vi "Teleop.vi"(10 "Match Info":T1={"Autonomous Elapsed Seconds"=0.0, "TeleOp Elapsed Seconds"=0.0, "Disabled Elapsed Seconds"=0.0, "Visited Autonomous"=FALSE, "Visited TeleOp"=FALSE, "Visited Disabled"=FALSE, "Autonomous Settings"={"Autonomous Style"=enum."Independent", "VI Refnum"=refnum}}, 11 "Call Context":T2) -> ()   [LabVIEW 2013]
doc: "This VI is called for each TeleOp packet received from the DS where the robot is not disabled. It is often used to read from the joysticks and update I/O or to update setpoints for timed control loops. It should complete and return within 20 milliseconds or it may miss DS packets."
uses:
  <vilib>/Rock Robotics/WPI/DriverStation/WPI_DriverStationDerivedRobotMode.ctl
  <vilib>/Rock Robotics/WPI/DriverStation/WPI_DriverStationMatch Info.ctl
  Robot Global Data.vi
  <vilib>/Rock Robotics/WPI/Joystick/WPI_JoystickGetSetRefNum.vi
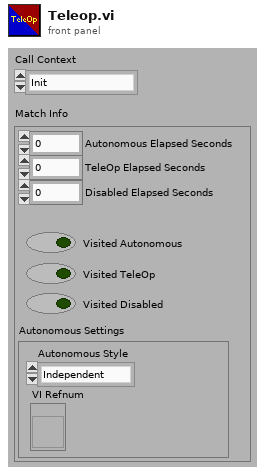
[diagram p1: front panel]
types:
  T1 = typedef "WPI_DriverStationMatch Info.ctl" = cluster{"Autonomous Elapsed Seconds":dbl, "TeleOp Elapsed Seconds":dbl, "Disabled Elapsed Seconds":dbl, "Visited Autonomous":bool, "Visited TeleOp":bool, "Visited Disabled":bool, "Autonomous Settings":cluster{"Autonomous Style":enum16{"Iterative", "Independent"}, "VI Refnum":refnum<vi>}}
  T2 = typedef "WPI_DriverStationDerivedRobotMode.ctl" = enum16{"Init", "Execute", "Stop"}
  T3 = typedef "WPI_JoystickDevRef.ctl" = cluster{"Device":T4}
  T4 = typedef "WPI_JoystickDeviceEnum.ctl" = enum16{"USB 1", "USB 2", "USB 3", "USB 4", "Kinect 1", "Kinect 2"}
  T5 = typedef "WPI_JoystickButtonState.ctl" = cluster{"Button 1":bool, "Button 2":bool, "Button 3":bool, "Button 4":bool, "Button 5":bool, "Button 6":bool, "Button 7":bool, "Button 8":bool, "Button 9":bool, "Button 10":bool, "Button 11":bool, "Button 12":bool}
  T6 = cluster{"axis 1 (x)":dbl, "axis 2 (y)":dbl, "axis 3 (throttle)":dbl, "axis 4":dbl, "axis 5":dbl, "axis 6":dbl}
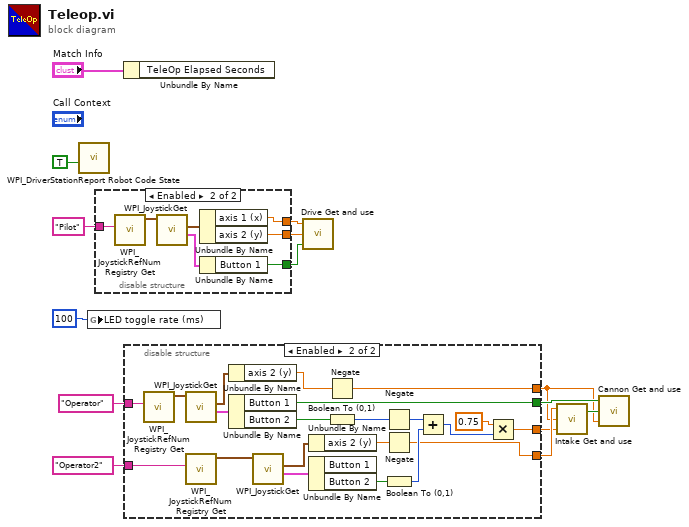
[diagram p0: block diagram]
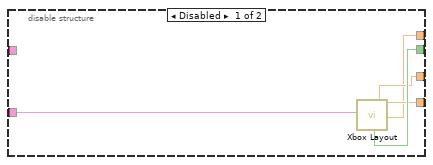
[diagram p2: hidden frame]
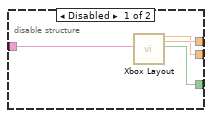
[diagram p3: hidden frame]
diagram:
  n1 = call <vilib>:"WPI_DriverStationReport Robot Code State.vi"("TeleOp"=TRUE ("Autonomous")) -> ()  [unwired: 10 in, 1 out]
  n2 = global write "Robot Global Data.vi" "LED toggle rate (ms)"(u32 100 ("LED ms toggle rate")) -> ()
  n3 = disable-structure shown="Enabled" {
    disable-tunnel: [w18 w20] -> w7
    disable-tunnel: [w17 w21] -> w6
    disable-tunnel: [w16 w19] -> w5
    disable-tunnel: "Pilot" ("refnum name") -> [w15 w25]
    frame Disabled {
      n4 = call "Xbox Layout.vi"("Joystick Name"=w15) -> ("Left Stick Y"=w17:dbl, "Left Stick X"=w18:dbl, "Left Stick Touch"=w16:bool)  [unwired: 3 in, 13 out]
    }
    frame Enabled {
      n5 = call <vilib>:"WPI_JoystickRefNum Registry Get.vi"("refnum name"=w25) -> ("JoystickDevRef"=w24:T3)  [unwired: 9 in, 1 out]
      n6 = call <vilib>:"WPI_JoystickGet.vi"("JoystickDevRef"=w24) -> ("Buttons"=w22:T5, "Axes"=w23:T6)  [unwired: 4 in, 1 out]
      n7 = Unbundle By Name(w23) -> ("axis 1 (x)"=w20:dbl, "axis 2 (y)"=w21:dbl)
      n8 = Unbundle By Name(w22) -> ("Button 1"=w19:bool)
    }
  }
  n9 = Unbundle By Name("Match Info") -> ()  [unwired: 1 out]
  n10 = disable-structure shown="Enabled" {
    disable-tunnel: "Operator2" ("refnum name") -> [w30 w50]
    disable-tunnel: [w29 w31] -> w10
    disable-tunnel: [w28 w40] -> w9
    disable-tunnel: [w27 w41] -> w8
    disable-tunnel: [w26 w35] -> w2
    disable-tunnel: "Operator" ("refnum name") -> [_ w39]
    frame Disabled {
      n11 = call "Xbox Layout.vi"("Joystick Name"=w30) -> ("X"=w29:bool, "L+R Throttles"=w27:dbl, "Left Stick Y"=w28:dbl, "Right Stick Y"=w26:dbl)  [unwired: 3 in, 12 out]
    }
    frame Enabled {
      n12 = call <vilib>:"WPI_JoystickRefNum Registry Get.vi"("refnum name"=w39) -> ("JoystickDevRef"=w38:T3)  [unwired: 9 in, 1 out]
      n13 = call <vilib>:"WPI_JoystickGet.vi"("JoystickDevRef"=w38) -> ("Buttons"=w34:T5, "Axes"=w37:T6)  [unwired: 4 in, 1 out]
      n14 = call <vilib>:"WPI_JoystickRefNum Registry Get.vi"("refnum name"=w50) -> ("JoystickDevRef"=w51:T3)  [unwired: 9 in, 1 out]
      n15 = Unbundle By Name(w37) -> ("axis 2 (y)"=w36:dbl)
      n16 = Unbundle By Name(w34) -> ("Button 1"=w31:bool, "Button 2"=w33:bool)
      n17 = call <vilib>:"WPI_JoystickGet.vi"("JoystickDevRef"=w51) -> ("Buttons"=w47:T5, "Axes"=w49:T6)  [unwired: 4 in, 1 out]
      n18 = Unbundle By Name(w49) -> ("axis 2 (y)"=w48:dbl)
      n19 = Unbundle By Name(w47) -> ("Button 2"=w32:bool)  [unwired: 1 out]
      n20 = Negate(x=w36) -> (-x=w35:dbl)
      n21 = Boolean To (0,1)(Boolean=w33) -> (0, 1=w42:i16)
      n22 = Negate(x=w42) -> (-x=w43:i16)
      n23 = Negate(x=w48) -> (-x=w40:dbl)
      n24 = Boolean To (0,1)(Boolean=w32) -> (0, 1=w44:i16)
      n25 = Add(x=w43, y=w44) -> (x+y=w46:i16)
      n26 = Multiply(x=0.75, y=w46) -> (x*y=w41:dbl)
    }
  }
  n27 = call "Drive Get and use.vi"("Slow Drive"=w5, "Y - Axis"=w6, "X - Axis"=w7) -> ()
  n28 = call "Intake Get and use.vi"("TakeBall"=w8, "Cannon vbus"=w2, "Upper Claw"=w9) -> ("InTake Max"=w4:bool)  [unwired: 1 out]
  n29 = call "Cannon Get and use.vi"("Move"=w2, "InTake Max"=w4, "Fire"=w10) -> ()  [unwired: 1 out]
